vi "RemoveWiringChangeImages.vi"(8 "error in (no error)":errorcluster, 11 "XML Path":path) -> (0 "error out":errorcluster)   [LabVIEW 2020]
panel:
  out "Array 2":string[](array[string])
  out "Deleted Files":path[](array[path])
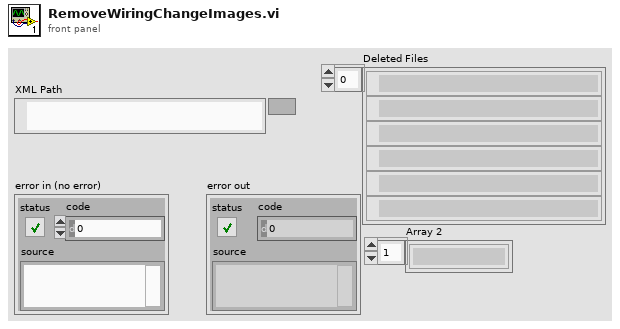
[diagram p1: front panel]
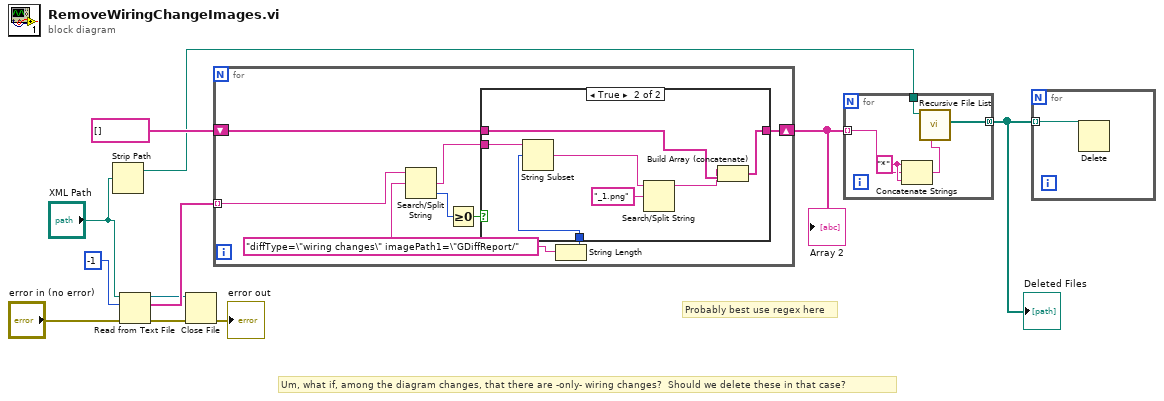
[diagram p0: block diagram]
diagram:
  # "Probably best use regex here"
  # "Um, what if, among the diagram changes, that there are -only- wiring changes?  Should we delete these in that case?"
  n1 = Strip Path(path="XML Path") -> (stripped path=w2:path)  [unwired: 1 out]
  n2 = Read from Text File(file (use dialog)="XML Path", count=-1, error in="error in (no error)") -> (refnum out=w6:refnum<file>, text=w10:string[], error out=w8:errorcluster)  [unwired: 1 in, 1 out]
  n3 = Close File(refnum=w6, error in=w8) -> (error out=→"error out":errorcluster)  [unwired: 1 out]
  n4 = for {
    tunnel: w10 -> [w16] mode=indexing
    shift-right: [w17] -> w3
    shift-left: string[] [] ("Array 2") -> [w18]
    w13 = "diffType=\"wiring changes\" imagePath1=\"GDiffReport/" ("search string")
    n5 = Search/Split String(string=w16, search string/char (-)=w13) -> (match + rest of string=w14:string, offset of match=w15:i32)  [unwired: 1 in, 1 out]
    n6 = Greater Or Equal To 0?(x=w15) -> (x >= 0?=w19:bool)
    n7 = String Length(string=w13) -> (length=w12:i32)
    n8 = case shown="True" w19 {
      tunnel: w14 -> [_ w23]
      tunnel: w18 -> [w20 w25]
      tunnel: [w20 w26] -> w17
      tunnel: w12 -> [_ w21]
      frame False {
      }
      frame True {
        n9 = String Subset(string=w23, offset (0)=w21) -> (substring=w22:string)  [unwired: 1 in]
        n10 = Search/Split String(string=w22, search string/char (-)="_1.png") -> (substring before match=w24:string)  [unwired: 1 in, 2 out]
        n11 = Build Array (concatenate)(w24, w25) -> (w26:string[])
      }
    }
  }
  "Array 2" <- w3
  n12 = for {
    tunnel: w3 -> [w29] mode=indexing
    tunnel: w2 -> [w32]
    tunnel: [w31] -> w1 mode=concatenating
    w30 = "*" ("string")
    n13 = Concatenate Strings(w30, w29, w30) -> (w28:string)
    n14 = call <vilib>:"Recursive File List.vi"("pattern"=w28, "Folder Path"=w32) -> ("All Files in Dir"=w31:path[])  [unwired: 5 in, 4 out]
  }
  "Deleted Files" <- w1
  n15 = for {
    tunnel: w1 -> [w33] mode=indexing
    n16 = Delete(path (use dialog)=w33) -> ()  [unwired: 4 in, 3 out]
  }
